vi "Lab Panel V5.25.vi"() -> ()   [LabVIEW 2017] (continued)
                      }
                      frame "CYCLE TEST" {
                      }
                      frame "T-RISE TEST" {
                      }
                    }
                    n1124 = Unbundle(w2151) -> ("CYCLE"=w2156:dbl)  [unwired: 2 out]
                    n1125 = Increment(x=w2148) -> (x+1=w2149:dbl)
                    n1126 = Greater Or Equal?(x=w2156, y=w2149) -> (x >= y?=w2158:bool)
                    n1127 = case shown="True" w2158 {
                      tunnel: w2153 -> [w2168 _]
                      tunnel: w2152 -> [w2167 _]
                      tunnel: w2151 -> [w2166 _]
                      tunnel: w2150 -> [w2165 _]
                      frame True {
                        n1128 = stacked-sequence {
                          tunnel: w2168 -> [w2172 _]
                          tunnel: w2167 -> [w2170 w2176]
                          tunnel: w2166 -> [_ w2179]
                          tunnel: w2165 -> [w2169 _]
                          frame #0 {
                            n1129 = Build Array(w2170) -> (w2173:string[])
                            n1130 = Build Array(w2172) -> (w2171:dbl[])
                            n1131 = TDMS Write(0:w2169, 5:"TEST PASS", 7:w2173, 9:w2171) -> (15:w2175:errorcluster)  [unwired: 2 in, 3 out]
                            n1132 = local write "data file error"(w2175) -> ()
                          }
                          frame #1 {
                            n1133 = Bundle(cluster=w2179, "STATUS"=w2176) -> (w2177:T4)  [unwired: 2 in]
                            n1134 = local write "RESULT LAB01-2"(TRUE) -> ()
                            n1135 = local write "DISP LAB01-2"(w2177) -> ()
                          }
                        }
                      }
                      frame False {
                      }
                    }
                  }
                }
              }
              frame #2 {
                # "LAB02-1"
                n1136 = Less?(x=w2180, y=2) -> (x < y?=w2183:bool)
                n1137 = local read "DISP LAB02-1"() -> (w2185:T4)
                n1138 = Unbundle(w2185) -> ("STATUS"=w2186:string)  [unwired: 2 out]
                n1139 = Equal?(x=w2186, y="RUN") -> (x = y?=w2182:bool)
                n1140 = And(x=w2182, y=w2183) -> (x .and. y?=w2181:bool)
                n1141 = case shown="True" w2181 {
                  tunnel: w2185 -> [_ w2191]
                  tunnel: w2180 -> [_ w2195]
                  frame False {
                  }
                  frame True {
                    n1142 = local read "TDMS LAB02-1"() -> (w2190:refnum<k34>)
                    n1143 = local read "SET LAB02-1"() -> (w2197:T5)
                    n1144 = Unbundle(w2191) -> ("CYCLE"=w2196:dbl)  [unwired: 2 out]
                    n1145 = Unbundle(w2197) -> ("CYCLES"=w2188:dbl, "T-RISE mins"=w2194:dbl)  [unwired: 3 out]
                    n1146 = case shown="\"T-RISE TEST\"" w2195 {
                      tunnel: w2194 -> [_ _ w2204]
                      tunnel: [w2199 w2201 w2204] -> w2193
                      tunnel: w2188 -> [w2199 w2201 _]
                      tunnel: ["CHART PASS" "CYCLE PASS" "T-RISE PASS"] -> w2192
                      frame "CHART TEST", Default {
                      }
                      frame "CYCLE TEST" {
                      }
                      frame "T-RISE TEST" {
                      }
                    }
                    n1147 = Increment(x=w2188) -> (x+1=w2189:dbl)
                    n1148 = Greater Or Equal?(x=w2196, y=w2189) -> (x >= y?=w2198:bool)
                    n1149 = case shown="True" w2198 {
                      tunnel: w2193 -> [w2208 _]
                      tunnel: w2192 -> [w2207 _]
                      tunnel: w2191 -> [w2206 _]
                      tunnel: w2190 -> [w2205 _]
                      frame True {
                        n1150 = stacked-sequence {
                          tunnel: w2208 -> [w2212 _]
                          tunnel: w2207 -> [w2210 w2216]
                          tunnel: w2206 -> [_ w2219]
                          tunnel: w2205 -> [w2209 _]
                          frame #0 {
                            n1151 = Build Array(w2210) -> (w2213:string[])
                            n1152 = Build Array(w2212) -> (w2211:dbl[])
                            n1153 = TDMS Write(0:w2209, 5:"TEST PASS", 7:w2213, 9:w2211) -> (15:w2215:errorcluster)  [unwired: 2 in, 3 out]
                            n1154 = local write "data file error"(w2215) -> ()
                          }
                          frame #1 {
                            n1155 = Bundle(cluster=w2219, "STATUS"=w2216) -> (w2217:T4)  [unwired: 2 in]
                            n1156 = local write "RESULT LAB02-1"(TRUE) -> ()
                            n1157 = local write "DISP LAB02-1"(w2217) -> ()
                          }
                        }
                      }
                      frame False {
                      }
                    }
                  }
                }
              }
              frame #3 {
                # "LAB02-2"
                n1158 = Less?(x=w2220, y=2) -> (x < y?=w2223:bool)
                n1159 = local read "DISP LAB02-2"() -> (w2225:T4)
                n1160 = Unbundle(w2225) -> ("STATUS"=w2226:string)  [unwired: 2 out]
                n1161 = Equal?(x=w2226, y="RUN") -> (x = y?=w2222:bool)
                n1162 = And(x=w2222, y=w2223) -> (x .and. y?=w2221:bool)
                n1163 = case shown="True" w2221 {
                  tunnel: w2225 -> [_ w2231]
                  tunnel: w2220 -> [_ w2235]
                  frame False {
                  }
                  frame True {
                    n1164 = local read "TDMS LAB02-2"() -> (w2230:refnum<k34>)
                    n1165 = local read "SET LAB02-2"() -> (w2237:T5)
                    n1166 = Unbundle(w2231) -> ("CYCLE"=w2236:dbl)  [unwired: 2 out]
                    n1167 = Unbundle(w2237) -> ("CYCLES"=w2228:dbl, "T-RISE mins"=w2234:dbl)  [unwired: 3 out]
                    n1168 = case shown="\"T-RISE TEST\"" w2235 {
                      tunnel: w2234 -> [_ _ w2244]
                      tunnel: [w2239 w2241 w2244] -> w2233
                      tunnel: w2228 -> [w2239 w2241 _]
                      tunnel: ["CHART PASS" "CYCLE PASS" "T-RISE PASS"] -> w2232
                      frame "CHART TEST", Default {
                      }
                      frame "CYCLE TEST" {
                      }
                      frame "T-RISE TEST" {
                      }
                    }
                    n1169 = Increment(x=w2228) -> (x+1=w2229:dbl)
                    n1170 = Greater Or Equal?(x=w2236, y=w2229) -> (x >= y?=w2238:bool)
                    n1171 = case shown="True" w2238 {
                      tunnel: w2233 -> [w2248 _]
                      tunnel: w2232 -> [w2247 _]
                      tunnel: w2231 -> [w2246 _]
                      tunnel: w2230 -> [w2245 _]
                      frame True {
                        n1172 = stacked-sequence {
                          tunnel: w2248 -> [w2252 _]
                          tunnel: w2247 -> [w2250 w2256]
                          tunnel: w2246 -> [_ w2259]
                          tunnel: w2245 -> [w2249 _]
                          frame #0 {
                            n1173 = Build Array(w2250) -> (w2253:string[])
                            n1174 = Build Array(w2252) -> (w2251:dbl[])
                            n1175 = TDMS Write(0:w2249, 5:"TEST PASS", 7:w2253, 9:w2251) -> (15:w2255:errorcluster)  [unwired: 2 in, 3 out]
                            n1176 = local write "data file error"(w2255) -> ()
                          }
                          frame #1 {
                            n1177 = Bundle(cluster=w2259, "STATUS"=w2256) -> (w2257:T4)  [unwired: 2 in]
                            n1178 = local write "RESULT LAB02-2"(TRUE) -> ()
                            n1179 = local write "DISP LAB02-2"(w2257) -> ()
                          }
                        }
                      }
                      frame False {
                      }
                    }
                  }
                }
              }
              frame #4 {
                # "LAB03-1"
                n1180 = Less?(x=w2260, y=2) -> (x < y?=w2263:bool)
                n1181 = local read "DISP LAB03-1"() -> (w2265:T4)
                n1182 = Unbundle(w2265) -> ("STATUS"=w2266:string)  [unwired: 2 out]
                n1183 = Equal?(x=w2266, y="RUN") -> (x = y?=w2262:bool)
                n1184 = And(x=w2262, y=w2263) -> (x .and. y?=w2261:bool)
                n1185 = case shown="True" w2261 {
                  tunnel: w2265 -> [_ w2271]
                  tunnel: w2260 -> [_ w2275]
                  frame False {
                  }
                  frame True {
                    n1186 = local read "TDMS LAB03-1"() -> (w2270:refnum<k34>)
                    n1187 = local read "SET LAB03-1"() -> (w2277:T5)
                    n1188 = Unbundle(w2271) -> ("CYCLE"=w2276:dbl)  [unwired: 2 out]
                    n1189 = Unbundle(w2277) -> ("CYCLES"=w2268:dbl, "T-RISE mins"=w2274:dbl)  [unwired: 3 out]
                    n1190 = case shown="\"T-RISE TEST\"" w2275 {
                      tunnel: w2274 -> [_ _ w2284]
                      tunnel: [w2279 w2281 w2284] -> w2273
                      tunnel: w2268 -> [w2279 w2281 _]
                      tunnel: ["CHART PASS" "CYCLE PASS" "T-RISE PASS"] -> w2272
                      frame "CHART TEST", Default {
                      }
                      frame "CYCLE TEST" {
                      }
                      frame "T-RISE TEST" {
                      }
                    }
                    n1191 = Increment(x=w2268) -> (x+1=w2269:dbl)
                    n1192 = Greater Or Equal?(x=w2276, y=w2269) -> (x >= y?=w2278:bool)
                    n1193 = case shown="True" w2278 {
                      tunnel: w2273 -> [w2288 _]
                      tunnel: w2272 -> [w2287 _]
                      tunnel: w2271 -> [w2286 _]
                      tunnel: w2270 -> [w2285 _]
                      frame True {
                        n1194 = stacked-sequence {
                          tunnel: w2288 -> [w2292 _]
                          tunnel: w2287 -> [w2290 w2296]
                          tunnel: w2286 -> [_ w2299]
                          tunnel: w2285 -> [w2289 _]
                          frame #0 {
                            n1195 = Build Array(w2290) -> (w2293:string[])
                            n1196 = Build Array(w2292) -> (w2291:dbl[])
                            n1197 = TDMS Write(0:w2289, 5:"TEST PASS", 7:w2293, 9:w2291) -> (15:w2295:errorcluster)  [unwired: 2 in, 3 out]
                            n1198 = local write "data file error"(w2295) -> ()
                          }
                          frame #1 {
                            n1199 = Bundle(cluster=w2299, "STATUS"=w2296) -> (w2297:T4)  [unwired: 2 in]
                            n1200 = local write "RESULT LAB03-1"(TRUE) -> ()
                            n1201 = local write "DISP LAB03-1"(w2297) -> ()
                          }
                        }
                      }
                      frame False {
                      }
                    }
                  }
                }
              }
              frame #5 {
                # "LAB03-2"
                n1202 = Less?(x=w2300, y=2) -> (x < y?=w2303:bool)
                n1203 = local read "DISP LAB03-2"() -> (w2305:T4)
                n1204 = Unbundle(w2305) -> ("STATUS"=w2306:string)  [unwired: 2 out]
                n1205 = Equal?(x=w2306, y="RUN") -> (x = y?=w2302:bool)
                n1206 = And(x=w2302, y=w2303) -> (x .and. y?=w2301:bool)
                n1207 = case shown="True" w2301 {
                  tunnel: w2305 -> [_ w2311]
                  tunnel: w2300 -> [_ w2315]
                  frame False {
                  }
                  frame True {
                    n1208 = local read "TDMS LAB03-2"() -> (w2310:refnum<k34>)
                    n1209 = local read "SET LAB03-2"() -> (w2317:T5)
                    n1210 = Unbundle(w2311) -> ("CYCLE"=w2316:dbl)  [unwired: 2 out]
                    n1211 = Unbundle(w2317) -> ("CYCLES"=w2308:dbl, "T-RISE mins"=w2314:dbl)  [unwired: 3 out]
                    n1212 = case shown="\"T-RISE TEST\"" w2315 {
                      tunnel: w2314 -> [_ _ w2324]
                      tunnel: [w2319 w2321 w2324] -> w2313
                      tunnel: w2308 -> [w2319 w2321 _]
                      tunnel: ["CHART PASS" "CYCLE PASS" "T-RISE PASS"] -> w2312
                      frame "CHART TEST", Default {
                      }
                      frame "CYCLE TEST" {
                      }
                      frame "T-RISE TEST" {
                      }
                    }
                    n1213 = Increment(x=w2308) -> (x+1=w2309:dbl)
                    n1214 = Greater Or Equal?(x=w2316, y=w2309) -> (x >= y?=w2318:bool)
                    n1215 = case shown="True" w2318 {
                      tunnel: w2313 -> [w2328 _]
                      tunnel: w2312 -> [w2327 _]
                      tunnel: w2311 -> [w2326 _]
                      tunnel: w2310 -> [w2325 _]
                      frame True {
                        n1216 = stacked-sequence {
                          tunnel: w2328 -> [w2332 _]
                          tunnel: w2327 -> [w2330 w2336]
                          tunnel: w2326 -> [_ w2339]
                          tunnel: w2325 -> [w2329 _]
                          frame #0 {
                            n1217 = Build Array(w2330) -> (w2333:string[])
                            n1218 = Build Array(w2332) -> (w2331:dbl[])
                            n1219 = TDMS Write(0:w2329, 5:"TEST PASS", 7:w2333, 9:w2331) -> (15:w2335:errorcluster)  [unwired: 2 in, 3 out]
                            n1220 = local write "data file error"(w2335) -> ()
                          }
                          frame #1 {
                            n1221 = Bundle(cluster=w2339, "STATUS"=w2336) -> (w2337:T4)  [unwired: 2 in]
                            n1222 = local write "RESULT LAB03-2"(TRUE) -> ()
                            n1223 = local write "DISP LAB03-2"(w2337) -> ()
                          }
                        }
                      }
                      frame False {
                      }
                    }
                  }
                }
              }
              frame #6 {
                # "LAB04-1"
                n1224 = Less?(x=w2340, y=2) -> (x < y?=w2343:bool)
                n1225 = local read "DISP LAB04-1"() -> (w2345:T4)
                n1226 = Unbundle(w2345) -> ("STATUS"=w2346:string)  [unwired: 2 out]
                n1227 = Equal?(x=w2346, y="RUN") -> (x = y?=w2342:bool)
                n1228 = And(x=w2342, y=w2343) -> (x .and. y?=w2341:bool)
                n1229 = case shown="True" w2341 {
                  tunnel: w2345 -> [_ w2351]
                  tunnel: w2340 -> [_ w2355]
                  frame False {
                  }
                  frame True {
                    n1230 = local read "TDMS LAB04-1"() -> (w2350:refnum<k34>)
                    n1231 = local read "SET LAB04-1"() -> (w2357:T5)
                    n1232 = Unbundle(w2351) -> ("CYCLE"=w2356:dbl)  [unwired: 2 out]
                    n1233 = Unbundle(w2357) -> ("CYCLES"=w2348:dbl, "T-RISE mins"=w2354:dbl)  [unwired: 3 out]
                    n1234 = case shown="\"T-RISE TEST\"" w2355 {
                      tunnel: w2354 -> [_ _ w2364]
                      tunnel: [w2359 w2361 w2364] -> w2353
                      tunnel: w2348 -> [w2359 w2361 _]
                      tunnel: ["CHART PASS" "CYCLE PASS" "T-RISE PASS"] -> w2352
                      frame "CHART TEST", Default {
                      }
                      frame "CYCLE TEST" {
                      }
                      frame "T-RISE TEST" {
                      }
                    }
                    n1235 = Increment(x=w2348) -> (x+1=w2349:dbl)
                    n1236 = Greater Or Equal?(x=w2356, y=w2349) -> (x >= y?=w2358:bool)
                    n1237 = case shown="True" w2358 {
                      tunnel: w2353 -> [w2368 _]
                      tunnel: w2352 -> [w2367 _]
                      tunnel: w2351 -> [w2366 _]
                      tunnel: w2350 -> [w2365 _]
                      frame True {
                        n1238 = stacked-sequence {
                          tunnel: w2368 -> [w2372 _]
                          tunnel: w2367 -> [w2370 w2376]
                          tunnel: w2366 -> [_ w2379]
                          tunnel: w2365 -> [w2369 _]
                          frame #0 {
                            n1239 = Build Array(w2370) -> (w2373:string[])
                            n1240 = Build Array(w2372) -> (w2371:dbl[])
                            n1241 = TDMS Write(0:w2369, 5:"TEST PASS", 7:w2373, 9:w2371) -> (15:w2375:errorcluster)  [unwired: 2 in, 3 out]
                            n1242 = local write "data file error"(w2375) -> ()
                          }
                          frame #1 {
                            n1243 = Bundle(cluster=w2379, "STATUS"=w2376) -> (w2377:T4)  [unwired: 2 in]
                            n1244 = local write "RESULT LAB04-1"(TRUE) -> ()
                            n1245 = local write "DISP LAB04-1"(w2377) -> ()
                          }
                        }
                      }
                      frame False {
                      }
                    }
                  }
                }
              }
              frame #7 {
                # "LAB04-2"
                n1246 = Less?(x=w2380, y=2) -> (x < y?=w2383:bool)
                n1247 = local read "DISP LAB04-2"() -> (w2385:T4)
                n1248 = Unbundle(w2385) -> ("STATUS"=w2386:string)  [unwired: 2 out]
                n1249 = Equal?(x=w2386, y="RUN") -> (x = y?=w2382:bool)
                n1250 = And(x=w2382, y=w2383) -> (x .and. y?=w2381:bool)
                n1251 = case shown="True" w2381 {
                  tunnel: w2385 -> [_ w2391]
                  tunnel: w2380 -> [_ w2395]
                  frame False {
                  }
                  frame True {
                    n1252 = local read "TDMS LAB04-2"() -> (w2390:refnum<k34>)
                    n1253 = local read "SET LAB04-2"() -> (w2397:T5)
                    n1254 = Unbundle(w2391) -> ("CYCLE"=w2396:dbl)  [unwired: 2 out]
                    n1255 = Unbundle(w2397) -> ("CYCLES"=w2388:dbl, "T-RISE mins"=w2394:dbl)  [unwired: 3 out]
                    n1256 = case shown="\"T-RISE TEST\"" w2395 {
                      tunnel: w2394 -> [_ _ w2404]
                      tunnel: [w2399 w2401 w2404] -> w2393
                      tunnel: w2388 -> [w2399 w2401 _]
                      tunnel: ["CHART PASS" "CYCLE PASS" "T-RISE PASS"] -> w2392
                      frame "CHART TEST", Default {
                      }
                      frame "CYCLE TEST" {
                      }
                      frame "T-RISE TEST" {
                      }
                    }
                    n1257 = Increment(x=w2388) -> (x+1=w2389:dbl)
                    n1258 = Greater Or Equal?(x=w2396, y=w2389) -> (x >= y?=w2398:bool)
                    n1259 = case shown="True" w2398 {
                      tunnel: w2393 -> [w2408 _]
                      tunnel: w2392 -> [w2407 _]
                      tunnel: w2391 -> [w2406 _]
                      tunnel: w2390 -> [w2405 _]
                      frame True {
                        n1260 = stacked-sequence {
                          tunnel: w2408 -> [w2412 _]
                          tunnel: w2407 -> [w2410 w2416]
                          tunnel: w2406 -> [_ w2419]
                          tunnel: w2405 -> [w2409 _]
                          frame #0 {
                            n1261 = Build Array(w2410) -> (w2413:string[])
                            n1262 = Build Array(w2412) -> (w2411:dbl[])
                            n1263 = TDMS Write(0:w2409, 5:"TEST PASS", 7:w2413, 9:w2411) -> (15:w2415:errorcluster)  [unwired: 2 in, 3 out]
                            n1264 = local write "data file error"(w2415) -> ()
                          }
                          frame #1 {
                            n1265 = Bundle(cluster=w2419, "STATUS"=w2416) -> (w2417:T4)  [unwired: 2 in]
                            n1266 = local write "RESULT LAB04-2"(TRUE) -> ()
                            n1267 = local write "DISP LAB04-2"(w2417) -> ()
                          }
                        }
                      }
                      frame False {
                      }
                    }
                  }
                }
              }
              frame #8 {
                # "LAB05-1"
                n1268 = Less?(x=w2420, y=2) -> (x < y?=w2423:bool)
                n1269 = local read "DISP LAB05-1"() -> (w2425:T4)
                n1270 = Unbundle(w2425) -> ("STATUS"=w2426:string)  [unwired: 2 out]
                n1271 = Equal?(x=w2426, y="RUN") -> (x = y?=w2422:bool)
                n1272 = And(x=w2422, y=w2423) -> (x .and. y?=w2421:bool)
                n1273 = case shown="True" w2421 {
                  tunnel: w2425 -> [_ w2431]
                  tunnel: w2420 -> [_ w2435]
                  frame False {
                  }
                  frame True {
                    n1274 = local read "TDMS LAB05-1"() -> (w2430:refnum<k34>)
                    n1275 = local read "SET LAB05-1"() -> (w2437:T5)
                    n1276 = Unbundle(w2431) -> ("CYCLE"=w2436:dbl)  [unwired: 2 out]
                    n1277 = Unbundle(w2437) -> ("CYCLES"=w2428:dbl, "T-RISE mins"=w2434:dbl)  [unwired: 3 out]
                    n1278 = case shown="\"T-RISE TEST\"" w2435 {
                      tunnel: w2434 -> [_ _ w2444]
                      tunnel: [w2439 w2441 w2444] -> w2433
                      tunnel: w2428 -> [w2439 w2441 _]
                      tunnel: ["CHART PASS" "CYCLE PASS" "T-RISE PASS"] -> w2432
                      frame "CHART TEST", Default {
                      }
                      frame "CYCLE TEST" {
                      }
                      frame "T-RISE TEST" {
                      }
                    }
                    n1279 = Increment(x=w2428) -> (x+1=w2429:dbl)
                    n1280 = Greater Or Equal?(x=w2436, y=w2429) -> (x >= y?=w2438:bool)
                    n1281 = case shown="True" w2438 {
                      tunnel: w2433 -> [w2448 _]
                      tunnel: w2432 -> [w2447 _]
                      tunnel: w2431 -> [w2446 _]
                      tunnel: w2430 -> [w2445 _]
                      frame True {
                        n1282 = stacked-sequence {
                          tunnel: w2448 -> [w2452 _]
                          tunnel: w2447 -> [w2450 w2456]
                          tunnel: w2446 -> [_ w2459]
                          tunnel: w2445 -> [w2449 _]
                          frame #0 {
                            n1283 = Build Array(w2450) -> (w2453:string[])
                            n1284 = Build Array(w2452) -> (w2451:dbl[])
                            n1285 = TDMS Write(0:w2449, 5:"TEST PASS", 7:w2453, 9:w2451) -> (15:w2455:errorcluster)  [unwired: 2 in, 3 out]
                            n1286 = local write "data file error"(w2455) -> ()
                          }
                          frame #1 {
                            n1287 = Bundle(cluster=w2459, "STATUS"=w2456) -> (w2457:T4)  [unwired: 2 in]
                            n1288 = local write "RESULT LAB05-1"(TRUE) -> ()
                            n1289 = local write "DISP LAB05-1"(w2457) -> ()
                          }
                        }
                      }
                      frame False {
                      }
                    }
                  }
                }
              }
              frame #9 {
                # "LAB05-2"
                n1290 = Less?(x=w2460, y=2) -> (x < y?=w2463:bool)
                n1291 = local read "DISP LAB05-2"() -> (w2465:T4)
                n1292 = Unbundle(w2465) -> ("STATUS"=w2466:string)  [unwired: 2 out]
                n1293 = Equal?(x=w2466, y="RUN") -> (x = y?=w2462:bool)
                n1294 = And(x=w2462, y=w2463) -> (x .and. y?=w2461:bool)
                n1295 = case shown="True" w2461 {
                  tunnel: w2465 -> [_ w2471]
                  tunnel: w2460 -> [_ w2475]
                  frame False {
                  }
                  frame True {
                    n1296 = local read "TDMS LAB05-2"() -> (w2470:refnum<k34>)
                    n1297 = local read "SET LAB05-2"() -> (w2477:T5)
                    n1298 = Unbundle(w2471) -> ("CYCLE"=w2476:dbl)  [unwired: 2 out]
                    n1299 = Unbundle(w2477) -> ("CYCLES"=w2468:dbl, "T-RISE mins"=w2474:dbl)  [unwired: 3 out]
                    n1300 = case shown="\"T-RISE TEST\"" w2475 {
                      tunnel: w2474 -> [_ _ w2484]
                      tunnel: [w2479 w2481 w2484] -> w2473
                      tunnel: w2468 -> [w2479 w2481 _]
                      tunnel: ["CHART PASS" "CYCLE PASS" "T-RISE PASS"] -> w2472
                      frame "CHART TEST", Default {
                      }
                      frame "CYCLE TEST" {
                      }
                      frame "T-RISE TEST" {
                      }
                    }
                    n1301 = Increment(x=w2468) -> (x+1=w2469:dbl)
                    n1302 = Greater Or Equal?(x=w2476, y=w2469) -> (x >= y?=w2478:bool)
                    n1303 = case shown="True" w2478 {
                      tunnel: w2473 -> [w2488 _]
                      tunnel: w2472 -> [w2487 _]
                      tunnel: w2471 -> [w2486 _]
                      tunnel: w2470 -> [w2485 _]
                      frame True {
                        n1304 = stacked-sequence {
                          tunnel: w2488 -> [w2492 _]
                          tunnel: w2487 -> [w2490 w2496]
                          tunnel: w2486 -> [_ w2499]
                          tunnel: w2485 -> [w2489 _]
                          frame #0 {
                            n1305 = Build Array(w2490) -> (w2493:string[])
                            n1306 = Build Array(w2492) -> (w2491:dbl[])
                            n1307 = TDMS Write(0:w2489, 5:"TEST PASS", 7:w2493, 9:w2491) -> (15:w2495:errorcluster)  [unwired: 2 in, 3 out]
                            n1308 = local write "data file error"(w2495) -> ()
                          }
                          frame #1 {
                            n1309 = Bundle(cluster=w2499, "STATUS"=w2496) -> (w2497:T4)  [unwired: 2 in]
                            n1310 = local write "RESULT LAB05-2"(TRUE) -> ()
                            n1311 = local write "DISP LAB05-2"(w2497) -> ()
                          }
                        }
                      }
                      frame False {
                      }
                    }
                  }
                }
              }
            }
          }
          frame #5 {
            # "check if test cycles reached for temperature rise test"
            n1312 = stacked-sequence {
              tunnel: w2529 -> [_ _ _ _ _ _ _ _ _ _]
              tunnel: w2528 -> [_ _ _ _ _ _ _ _ _ _]
              tunnel: w2527 -> [_ _ _ _ _ _ _ _ _ _]
              tunnel: w2526 -> [_ _ _ _ _ _ _ _ _ _]
              tunnel: w2525 -> [_ _ _ _ _ _ _ _ _ _]
              tunnel: w2524 -> [_ _ _ _ _ _ _ _ _ _]
              tunnel: w2523 -> [_ _ _ _ _ _ _ _ _ _]
              tunnel: w2522 -> [_ _ _ _ _ _ _ _ _ _]
              tunnel: w2521 -> [_ _ _ _ _ _ _ _ _ _]
              tunnel: w2520 -> [_ _ _ _ _ _ _ _ _ _]
              tunnel: w2519 -> [w2535 _ _ _ _ _ _ _ _ _]
              tunnel: w2509 -> [w2530 _ _ _ _ _ _ _ _ _]
              tunnel: w2518 -> [_ w2561 _ _ _ _ _ _ _ _]
              tunnel: w2517 -> [_ _ w2591 _ _ _ _ _ _ _]
              tunnel: w2516 -> [_ _ _ w2621 _ _ _ _ _ _]
              tunnel: w2515 -> [_ _ _ _ w2651 _ _ _ _ _]
              tunnel: w2514 -> [_ _ _ _ _ w2681 _ _ _ _]
              tunnel: w2513 -> [_ _ _ _ _ _ w2711 _ _ _]
              tunnel: w2512 -> [_ _ _ _ _ _ _ w2741 _ _]
              tunnel: w2511 -> [_ _ _ _ _ _ _ _ w2771 _]
              tunnel: w2510 -> [_ _ _ _ _ _ _ _ _ w2801]
              tunnel: w2508 -> [_ w2560 _ _ _ _ _ _ _ _]
              tunnel: w2507 -> [_ _ w2590 _ _ _ _ _ _ _]
              tunnel: w2506 -> [_ _ _ w2620 _ _ _ _ _ _]
              tunnel: w2505 -> [_ _ _ _ w2650 _ _ _ _ _]
              tunnel: w2504 -> [_ _ _ _ _ w2680 _ _ _ _]
              tunnel: w2503 -> [_ _ _ _ _ _ w2710 _ _ _]
              tunnel: w2502 -> [_ _ _ _ _ _ _ w2740 _ _]
              tunnel: w2501 -> [_ _ _ _ _ _ _ _ w2770 _]
              tunnel: w2500 -> [_ _ _ _ _ _ _ _ _ w2800]
              frame #0 {
                # "LAB01-1"
                n1313 = Equal?(x=w2535, y=2) -> (x = y?=w2533:bool)
                n1314 = local read "DISP LAB01-1"() -> (w2536:T4)
                n1315 = Unbundle(w2536) -> ("STATUS"=w2537:string)  [unwired: 2 out]
                n1316 = Equal?(x=w2537, y="RUN") -> (x = y?=w2532:bool)
                n1317 = And(x=w2532, y=w2533) -> (x .and. y?=w2531:bool)
                n1318 = case shown="True" w2531 {
                  tunnel: w2536 -> [_ w2540]
                  tunnel: w2530 -> [_ w2543]
                  frame False {
                  }
                  frame True {
                    n1319 = local read "SET LAB01-1"() -> (w2542:T5)
                    n1320 = local read "TDMS LAB01-1"() -> (w2539:refnum<k34>)
                    n1321 = Unbundle(w2540) -> ("CYCLE"=w2544:dbl)  [unwired: 2 out]
                    n1322 = Unbundle(w2542) -> ("T-RISE mins"=w2541:dbl)  [unwired: 4 out]
                    n1323 = Greater Or Equal?(x=w2544, y=w2543) -> (x >= y?=w2545:bool)
                    n1324 = case shown="True" w2545 {
                      tunnel: w2541 -> [w2548 _]
                      tunnel: w2540 -> [w2547 _]
                      tunnel: w2539 -> [w2546 _]
                      frame True {
                        n1325 = stacked-sequence {
                          tunnel: w2548 -> [w2551 _]
                          tunnel: w2547 -> [_ w2556]
                          tunnel: w2546 -> [w2549 _]
                          frame #0 {
                            n1326 = Build Array("T-RISE") -> (w2553:string[])
                            n1327 = Build Array(w2551) -> (w2552:dbl[])
                            n1328 = TDMS Write(0:w2549, 5:"TEST PASS", 7:w2553, 9:w2552) -> (15:w2555:errorcluster)  [unwired: 2 in, 3 out]
                            n1329 = local write "data file error"(w2555) -> ()
                          }
                          frame #1 {
                            n1330 = Bundle(cluster=w2556, "STATUS"="T-RISE PASS") -> (w2558:T4)  [unwired: 2 in]
                            n1331 = local write "RESULT LAB01-1"(TRUE) -> ()
                            n1332 = local write "DISP LAB01-1"(w2558) -> ()
                          }
                        }
                      }
                      frame False {
                      }
                    }
                  }
                }
              }
              frame #1 {
                # "LAB01-2"
                n1333 = Equal?(x=w2561, y=2) -> (x = y?=w2564:bool)
                n1334 = local read "DISP LAB01-2"() -> (w2566:T4)
                n1335 = Unbundle(w2566) -> ("STATUS"=w2567:string)  [unwired: 2 out]
                n1336 = Equal?(x=w2567, y="RUN") -> (x = y?=w2563:bool)
                n1337 = And(x=w2563, y=w2564) -> (x .and. y?=w2562:bool)
                n1338 = case shown="True" w2562 {
                  tunnel: w2566 -> [_ w2570]
                  tunnel: w2560 -> [_ w2573]
                  frame False {
                  }
                  frame True {
                    n1339 = local read "SET LAB01-2"() -> (w2572:T5)
                    n1340 = local read "TDMS LAB01-2"() -> (w2569:refnum<k34>)
                    n1341 = Unbundle(w2570) -> ("CYCLE"=w2574:dbl)  [unwired: 2 out]
                    n1342 = Unbundle(w2572) -> ("T-RISE mins"=w2571:dbl)  [unwired: 4 out]
                    n1343 = Greater Or Equal?(x=w2574, y=w2573) -> (x >= y?=w2575:bool)
                    n1344 = case shown="True" w2575 {
                      tunnel: w2571 -> [w2578 _]
                      tunnel: w2570 -> [w2577 _]
                      tunnel: w2569 -> [w2576 _]
                      frame True {
                        n1345 = stacked-sequence {
                          tunnel: w2578 -> [w2581 _]
                          tunnel: w2577 -> [_ w2586]
                          tunnel: w2576 -> [w2579 _]
                          frame #0 {
                            n1346 = Build Array("T-RISE") -> (w2583:string[])
                            n1347 = Build Array(w2581) -> (w2582:dbl[])
                            n1348 = TDMS Write(0:w2579, 5:"TEST PASS", 7:w2583, 9:w2582) -> (15:w2585:errorcluster)  [unwired: 2 in, 3 out]
                            n1349 = local write "data file error"(w2585) -> ()
                          }
                          frame #1 {
                            n1350 = Bundle(cluster=w2586, "STATUS"="T-RISE PASS") -> (w2588:T4)  [unwired: 2 in]
                            n1351 = local write "RESULT LAB01-2"(TRUE) -> ()
                            n1352 = local write "DISP LAB01-2"(w2588) -> ()
                          }
                        }
                      }
                      frame False {
                      }
                    }
                  }
                }
              }
              frame #2 {
                # "LAB02-1"
                n1353 = Equal?(x=w2591, y=2) -> (x = y?=w2594:bool)
                n1354 = local read "DISP LAB02-1"() -> (w2596:T4)
                n1355 = Unbundle(w2596) -> ("STATUS"=w2597:string)  [unwired: 2 out]
                n1356 = Equal?(x=w2597, y="RUN") -> (x = y?=w2593:bool)
                n1357 = And(x=w2593, y=w2594) -> (x .and. y?=w2592:bool)
                n1358 = case shown="True" w2592 {
                  tunnel: w2596 -> [_ w2600]
                  tunnel: w2590 -> [_ w2603]
                  frame False {
                  }
                  frame True {
                    n1359 = local read "SET LAB02-1"() -> (w2602:T5)
                    n1360 = local read "TDMS LAB02-1"() -> (w2599:refnum<k34>)
                    n1361 = Unbundle(w2600) -> ("CYCLE"=w2604:dbl)  [unwired: 2 out]
                    n1362 = Unbundle(w2602) -> ("T-RISE mins"=w2601:dbl)  [unwired: 4 out]
                    n1363 = Greater Or Equal?(x=w2604, y=w2603) -> (x >= y?=w2605:bool)
                    n1364 = case shown="True" w2605 {
                      tunnel: w2601 -> [w2608 _]
                      tunnel: w2600 -> [w2607 _]
                      tunnel: w2599 -> [w2606 _]
                      frame True {
                        n1365 = stacked-sequence {
                          tunnel: w2608 -> [w2611 _]
                          tunnel: w2607 -> [_ w2616]
                          tunnel: w2606 -> [w2609 _]
                          frame #0 {
                            n1366 = Build Array("T-RISE") -> (w2613:string[])
                            n1367 = Build Array(w2611) -> (w2612:dbl[])
                            n1368 = TDMS Write(0:w2609, 5:"TEST PASS", 7:w2613, 9:w2612) -> (15:w2615:errorcluster)  [unwired: 2 in, 3 out]
                            n1369 = local write "data file error"(w2615) -> ()
                          }
                          frame #1 {
                            n1370 = Bundle(cluster=w2616, "STATUS"="T-RISE PASS") -> (w2618:T4)  [unwired: 2 in]
                            n1371 = local write "RESULT LAB02-1"(TRUE) -> ()
                            n1372 = local write "DISP LAB02-1"(w2618) -> ()
                          }
                        }
                      }
                      frame False {
                      }
                    }
                  }
                }
              }
              frame #3 {
                # "LAB02-2"
                n1373 = Equal?(x=w2621, y=2) -> (x = y?=w2624:bool)
                n1374 = local read "DISP LAB02-2"() -> (w2626:T4)
                n1375 = Unbundle(w2626) -> ("STATUS"=w2627:string)  [unwired: 2 out]
                n1376 = Equal?(x=w2627, y="RUN") -> (x = y?=w2623:bool)
                n1377 = And(x=w2623, y=w2624) -> (x .and. y?=w2622:bool)
                n1378 = case shown="True" w2622 {
                  tunnel: w2626 -> [_ w2630]
                  tunnel: w2620 -> [_ w2633]
                  frame False {
                  }
                  frame True {
                    n1379 = local read "SET LAB02-2"() -> (w2632:T5)
                    n1380 = local read "TDMS LAB02-2"() -> (w2629:refnum<k34>)
                    n1381 = Unbundle(w2630) -> ("CYCLE"=w2634:dbl)  [unwired: 2 out]
                    n1382 = Unbundle(w2632) -> ("T-RISE mins"=w2631:dbl)  [unwired: 4 out]
                    n1383 = Greater Or Equal?(x=w2634, y=w2633) -> (x >= y?=w2635:bool)
                    n1384 = case shown="True" w2635 {
                      tunnel: w2631 -> [w2638 _]
                      tunnel: w2630 -> [w2637 _]
                      tunnel: w2629 -> [w2636 _]
                      frame True {
                        n1385 = stacked-sequence {
                          tunnel: w2638 -> [w2641 _]
                          tunnel: w2637 -> [_ w2646]
                          tunnel: w2636 -> [w2639 _]
                          frame #0 {
                            n1386 = Build Array("T-RISE") -> (w2643:string[])
                            n1387 = Build Array(w2641) -> (w2642:dbl[])
                            n1388 = TDMS Write(0:w2639, 5:"TEST PASS", 7:w2643, 9:w2642) -> (15:w2645:errorcluster)  [unwired: 2 in, 3 out]
                            n1389 = local write "data file error"(w2645) -> ()
                          }
                          frame #1 {
                            n1390 = Bundle(cluster=w2646, "STATUS"="T-RISE PASS") -> (w2648:T4)  [unwired: 2 in]
                            n1391 = local write "RESULT LAB02-2"(TRUE) -> ()
                            n1392 = local write "DISP LAB02-2"(w2648) -> ()
                          }
                        }
                      }
                      frame False {
                      }
                    }
                  }
                }
              }
              frame #4 {
                # "LAB03-1"
                n1393 = Equal?(x=w2651, y=2) -> (x = y?=w2654:bool)
                n1394 = local read "DISP LAB03-1"() -> (w2656:T4)
                n1395 = Unbundle(w2656) -> ("STATUS"=w2657:string)  [unwired: 2 out]
                n1396 = Equal?(x=w2657, y="RUN") -> (x = y?=w2653:bool)
                n1397 = And(x=w2653, y=w2654) -> (x .and. y?=w2652:bool)
                n1398 = case shown="True" w2652 {
                  tunnel: w2656 -> [_ w2660]
                  tunnel: w2650 -> [_ w2663]
                  frame False {
                  }
                  frame True {
                    n1399 = local read "SET LAB03-1"() -> (w2662:T5)
                    n1400 = local read "TDMS LAB03-1"() -> (w2659:refnum<k34>)
                    n1401 = Unbundle(w2660) -> ("CYCLE"=w2664:dbl)  [unwired: 2 out]
                    n1402 = Unbundle(w2662) -> ("T-RISE mins"=w2661:dbl)  [unwired: 4 out]
                    n1403 = Greater Or Equal?(x=w2664, y=w2663) -> (x >= y?=w2665:bool)
                    n1404 = case shown="True" w2665 {
                      tunnel: w2661 -> [w2668 _]
                      tunnel: w2660 -> [w2667 _]
                      tunnel: w2659 -> [w2666 _]
                      frame True {
                        n1405 = stacked-sequence {
                          tunnel: w2668 -> [w2671 _]
                          tunnel: w2667 -> [_ w2676]
                          tunnel: w2666 -> [w2669 _]
                          frame #0 {
                            n1406 = Build Array("T-RISE") -> (w2673:string[])
                            n1407 = Build Array(w2671) -> (w2672:dbl[])
                            n1408 = TDMS Write(0:w2669, 5:"TEST PASS", 7:w2673, 9:w2672) -> (15:w2675:errorcluster)  [unwired: 2 in, 3 out]
                            n1409 = local write "data file error"(w2675) -> ()
                          }
                          frame #1 {
                            n1410 = Bundle(cluster=w2676, "STATUS"="T-RISE PASS") -> (w2678:T4)  [unwired: 2 in]
                            n1411 = local write "RESULT LAB03-1"(TRUE) -> ()
                            n1412 = local write "DISP LAB03-1"(w2678) -> ()
                          }
                        }
                      }
                      frame False {
                      }
                    }
                  }
                }
              }
              frame #5 {
                # "LAB03-2"
                n1413 = Equal?(x=w2681, y=2) -> (x = y?=w2684:bool)
                n1414 = local read "DISP LAB03-2"() -> (w2686:T4)
                n1415 = Unbundle(w2686) -> ("STATUS"=w2687:string)  [unwired: 2 out]
                n1416 = Equal?(x=w2687, y="RUN") -> (x = y?=w2683:bool)
                n1417 = And(x=w2683, y=w2684) -> (x .and. y?=w2682:bool)
                n1418 = case shown="True" w2682 {
                  tunnel: w2686 -> [_ w2690]
                  tunnel: w2680 -> [_ w2693]
                  frame False {
                  }
                  frame True {
                    n1419 = local read "SET LAB03-2"() -> (w2692:T5)
                    n1420 = local read "TDMS LAB03-2"() -> (w2689:refnum<k34>)
                    n1421 = Unbundle(w2690) -> ("CYCLE"=w2694:dbl)  [unwired: 2 out]
                    n1422 = Unbundle(w2692) -> ("T-RISE mins"=w2691:dbl)  [unwired: 4 out]
                    n1423 = Greater Or Equal?(x=w2694, y=w2693) -> (x >= y?=w2695:bool)
                    n1424 = case shown="True" w2695 {
                      tunnel: w2691 -> [w2698 _]
                      tunnel: w2690 -> [w2697 _]
                      tunnel: w2689 -> [w2696 _]
                      frame True {
                        n1425 = stacked-sequence {
                          tunnel: w2698 -> [w2701 _]
                          tunnel: w2697 -> [_ w2706]
                          tunnel: w2696 -> [w2699 _]
                          frame #0 {
                            n1426 = Build Array("T-RISE") -> (w2703:string[])
                            n1427 = Build Array(w2701) -> (w2702:dbl[])
                            n1428 = TDMS Write(0:w2699, 5:"TEST PASS", 7:w2703, 9:w2702) -> (15:w2705:errorcluster)  [unwired: 2 in, 3 out]
                            n1429 = local write "data file error"(w2705) -> ()
                          }
                          frame #1 {
                            n1430 = Bundle(cluster=w2706, "STATUS"="T-RISE PASS") -> (w2708:T4)  [unwired: 2 in]
                            n1431 = local write "RESULT LAB03-2"(TRUE) -> ()
                            n1432 = local write "DISP LAB03-2"(w2708) -> ()
                          }
                        }
                      }
                      frame False {
                      }
                    }
                  }
                }
              }
              frame #6 {
                # "LAB04-1"
                n1433 = Equal?(x=w2711, y=2) -> (x = y?=w2714:bool)
                n1434 = local read "DISP LAB04-1"() -> (w2716:T4)
                n1435 = Unbundle(w2716) -> ("STATUS"=w2717:string)  [unwired: 2 out]
                n1436 = Equal?(x=w2717, y="RUN") -> (x = y?=w2713:bool)
                n1437 = And(x=w2713, y=w2714) -> (x .and. y?=w2712:bool)
                n1438 = case shown="True" w2712 {
                  tunnel: w2716 -> [_ w2720]
                  tunnel: w2710 -> [_ w2723]
                  frame False {
                  }
                  frame True {
                    n1439 = local read "SET LAB04-1"() -> (w2722:T5)
                    n1440 = local read "TDMS LAB04-1"() -> (w2719:refnum<k34>)
                    n1441 = Unbundle(w2720) -> ("CYCLE"=w2724:dbl)  [unwired: 2 out]
                    n1442 = Unbundle(w2722) -> ("T-RISE mins"=w2721:dbl)  [unwired: 4 out]
                    n1443 = Greater Or Equal?(x=w2724, y=w2723) -> (x >= y?=w2725:bool)
                    n1444 = case shown="True" w2725 {
                      tunnel: w2721 -> [w2728 _]
                      tunnel: w2720 -> [w2727 _]
                      tunnel: w2719 -> [w2726 _]
                      frame True {
                        n1445 = stacked-sequence {
                          tunnel: w2728 -> [w2731 _]
                          tunnel: w2727 -> [_ w2736]
                          tunnel: w2726 -> [w2729 _]
                          frame #0 {
                            n1446 = Build Array("T-RISE") -> (w2733:string[])
                            n1447 = Build Array(w2731) -> (w2732:dbl[])
                            n1448 = TDMS Write(0:w2729, 5:"TEST PASS", 7:w2733, 9:w2732) -> (15:w2735:errorcluster)  [unwired: 2 in, 3 out]
                            n1449 = local write "data file error"(w2735) -> ()
                          }
                          frame #1 {
                            n1450 = Bundle(cluster=w2736, "STATUS"="T-RISE PASS") -> (w2738:T4)  [unwired: 2 in]
                            n1451 = local write "RESULT LAB04-1"(TRUE) -> ()
                            n1452 = local write "DISP LAB04-1"(w2738) -> ()
                          }
                        }
                      }
                      frame False {
                      }
                    }
                  }
                }
              }
              frame #7 {
                # "LAB04-2"
                n1453 = Equal?(x=w2741, y=2) -> (x = y?=w2744:bool)
                n1454 = local read "DISP LAB04-2"() -> (w2746:T4)
                n1455 = Unbundle(w2746) -> ("STATUS"=w2747:string)  [unwired: 2 out]
                n1456 = Equal?(x=w2747, y="RUN") -> (x = y?=w2743:bool)
                n1457 = And(x=w2743, y=w2744) -> (x .and. y?=w2742:bool)
                n1458 = case shown="True" w2742 {
                  tunnel: w2746 -> [_ w2750]
                  tunnel: w2740 -> [_ w2753]
                  frame False {
                  }
                  frame True {
                    n1459 = local read "SET LAB04-2"() -> (w2752:T5)
                    n1460 = local read "TDMS LAB04-2"() -> (w2749:refnum<k34>)
                    n1461 = Unbundle(w2750) -> ("CYCLE"=w2754:dbl)  [unwired: 2 out]
                    n1462 = Unbundle(w2752) -> ("T-RISE mins"=w2751:dbl)  [unwired: 4 out]
                    n1463 = Greater Or Equal?(x=w2754, y=w2753) -> (x >= y?=w2755:bool)
                    n1464 = case shown="True" w2755 {
                      tunnel: w2751 -> [w2758 _]
                      tunnel: w2750 -> [w2757 _]
                      tunnel: w2749 -> [w2756 _]
                      frame True {
                        n1465 = stacked-sequence {
                          tunnel: w2758 -> [w2761 _]
                          tunnel: w2757 -> [_ w2766]
                          tunnel: w2756 -> [w2759 _]
                          frame #0 {
                            n1466 = Build Array("T-RISE") -> (w2763:string[])
                            n1467 = Build Array(w2761) -> (w2762:dbl[])
                            n1468 = TDMS Write(0:w2759, 5:"TEST PASS", 7:w2763, 9:w2762) -> (15:w2765:errorcluster)  [unwired: 2 in, 3 out]
                            n1469 = local write "data file error"(w2765) -> ()
                          }
                          frame #1 {
                            n1470 = Bundle(cluster=w2766, "STATUS"="T-RISE PASS") -> (w2768:T4)  [unwired: 2 in]
                            n1471 = local write "RESULT LAB04-2"(TRUE) -> ()
                            n1472 = local write "DISP LAB04-2"(w2768) -> ()
                          }
                        }
                      }
                      frame False {
                      }
                    }
                  }
                }
              }
              frame #8 {
                # "LAB05-1"
                n1473 = Equal?(x=w2771, y=2) -> (x = y?=w2774:bool)
                n1474 = local read "DISP LAB05-1"() -> (w2776:T4)
                n1475 = Unbundle(w2776) -> ("STATUS"=w2777:string)  [unwired: 2 out]
                n1476 = Equal?(x=w2777, y="RUN") -> (x = y?=w2773:bool)
                n1477 = And(x=w2773, y=w2774) -> (x .and. y?=w2772:bool)
                n1478 = case shown="True" w2772 {
                  tunnel: w2776 -> [_ w2780]
                  tunnel: w2770 -> [_ w2783]
                  frame False {
                  }
                  frame True {
                    n1479 = local read "SET LAB05-1"() -> (w2782:T5)
                    n1480 = local read "TDMS LAB05-1"() -> (w2779:refnum<k34>)
                    n1481 = Unbundle(w2780) -> ("CYCLE"=w2784:dbl)  [unwired: 2 out]
                    n1482 = Unbundle(w2782) -> ("T-RISE mins"=w2781:dbl)  [unwired: 4 out]
                    n1483 = Greater Or Equal?(x=w2784, y=w2783) -> (x >= y?=w2785:bool)
                    n1484 = case shown="True" w2785 {
                      tunnel: w2781 -> [w2788 _]
                      tunnel: w2780 -> [w2787 _]
                      tunnel: w2779 -> [w2786 _]
                      frame True {
